vi "ExSubCreateFileImage.vi"(2 "error in (no error)":errorcluster, 3 "File  Name":string, 5 "Camera Handle":u32) -> (0 "error out":errorcluster, 1 "Handles Out":T1)   [LabVIEW 2010]
panel:
  # "ExSubCreateFileImage:\nThis is a SubVI that creates a file, and image \nobjects and returns the handles bundled in a cluster \nthat includes a pulser and camera handle"
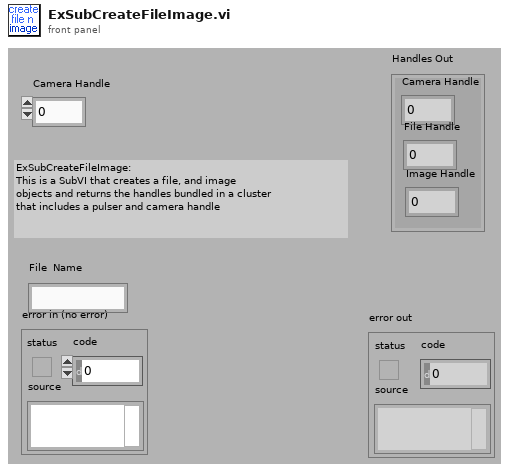
[diagram p1: front panel]
types:
  T1 = cluster{"Camera Handle":u32, "File Handle":u32, "Image Handle":u32}
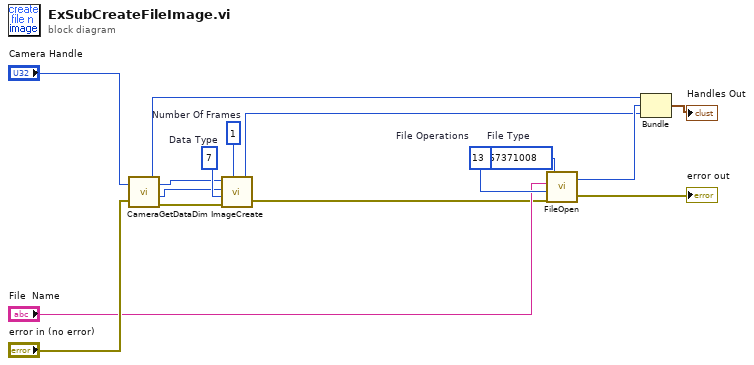
[diagram p0: block diagram]
diagram:
  w5 = u32 1  # Number Of Frames
  w6 = u32 7  # Data Type
  w8 = 13  # File Operations
  w9 = 67371008  # File Type
  n1 = call <userlib>:"CameraGetDataDim.vi"("Camera Handle"="Camera Handle", "error in"="error in (no error)") -> ("Camera Handle"=w12:u32, "Xdim"=w3:u32, "Ydim"=w4:u32, "error out"=w16:errorcluster)
  n2 = call <userlib>:"ImageCreate.vi"("X dimension"=w3, "Y dimension"=w4, "Data Type"=w6, "error in"=w16, "Number Of Frames"=w5) -> ("Image Handle"=w10:u32, "error out"=w1:errorcluster)
  n3 = call <userlib>:"FileOpen.vi"("error in"=w1, "File Operations"=w8, "FileName"="File  Name", "File Type"=w9) -> ("error out"=→"error out":errorcluster, "File Handle"=w11:u32)
  n4 = Bundle("Camera Handle"=w12, "File Handle"=w11, "Image Handle"=w10) -> (→"Handles Out":T1)  [unwired: 1 in]
